vi "ControlShooter.vi"(1 "State":T2) -> (0 "To Shooter\nSolenoid Loop":T1=enum."Forward")   [LabVIEW 2013]
uses:
  typedefs/subStates.ctl
  <vilib>/Rock Robotics/WPI/Solenoid/WPI_SolenoidValue.ctl
  typedefs/fg_typedef.ctl
  <vilib>/Rock Robotics/WPI/Solenoid/WPI_SolenoidGetEnum.vi
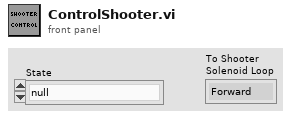
[diagram p1: front panel]
types:
  T1 = typedef "WPI_SolenoidValue.ctl" = enum16{"Off", "On", "Forward", "Reverse"}
  T2 = typedef "subStates.ctl" = enum16{"null", "wait", "driver control", "auto", "manual override", "hold position", "rotate", "pickup", "pass", "load", "goto shoot", "shoot", "cancel", "end"}
  T3 = typedef "fg_typedef.ctl" = enum16{"Get", "Set"}
  T4 = typedef "WPI_DigitalInputDevRef.ctl" = cluster{"DevStatus":errorcluster, "DIO Channel":T5, "Digital Module":T6}
  T5 = typedef "FPGA_DIOChannel.ctl" = enum8{"DIO 1", "DIO 2", "DIO 3", "DIO 4", "DIO 5", "DIO 6", "DIO 7", "DIO 8", "DIO 9", "DIO 10", "DIO 11", "DIO 12", "DIO 13", "DIO 14", "Invalid"}
  T6 = typedef "FPGA_TypedefDigitalModule.ctl" = enum16{"Digital Module 1", "Digital Module 2"}
  T7 = typedef "WPI_SolenoidDevRef.ctl" = cluster{"DevStatus":errorcluster, "Solenoid Module":T8, "Forward Solenoid Channel":T9, "Reverse Solenoid Channel":T9}
  T8 = typedef "FPGA_TypedefSolenoidModule.ctl" = enum16{"Solenoid Module 1", "Solenoid Module 2"}
  T9 = typedef "WPI_SolenoidChannel.ctl" = enum8{"Solenoid 1", "Solenoid 2", "Solenoid 3", "Solenoid 4", "Solenoid 5", "Solenoid 6", "Solenoid 7", "Solenoid 8", "Invalid"}
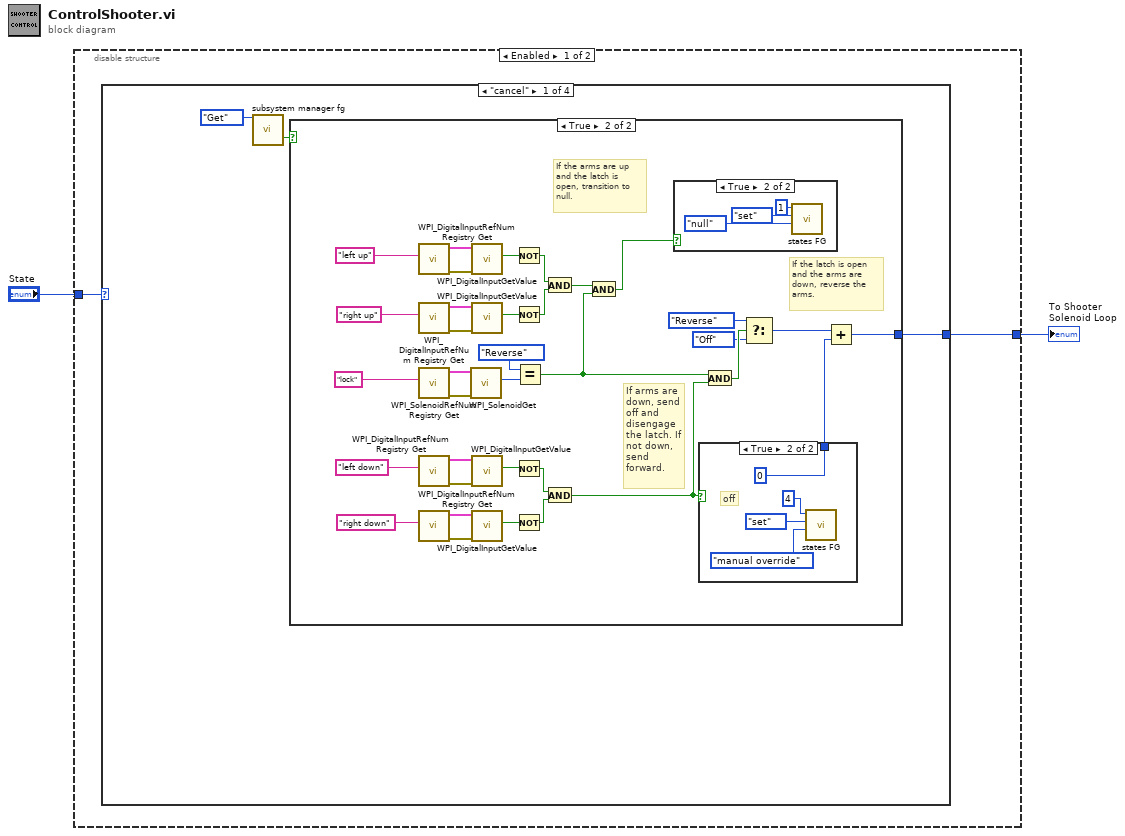
[diagram p0: block diagram]
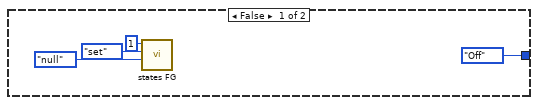
[diagram p2: hidden frame]
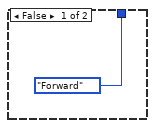
[diagram p4: hidden frame]
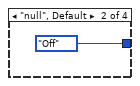
[diagram p5: hidden frame]
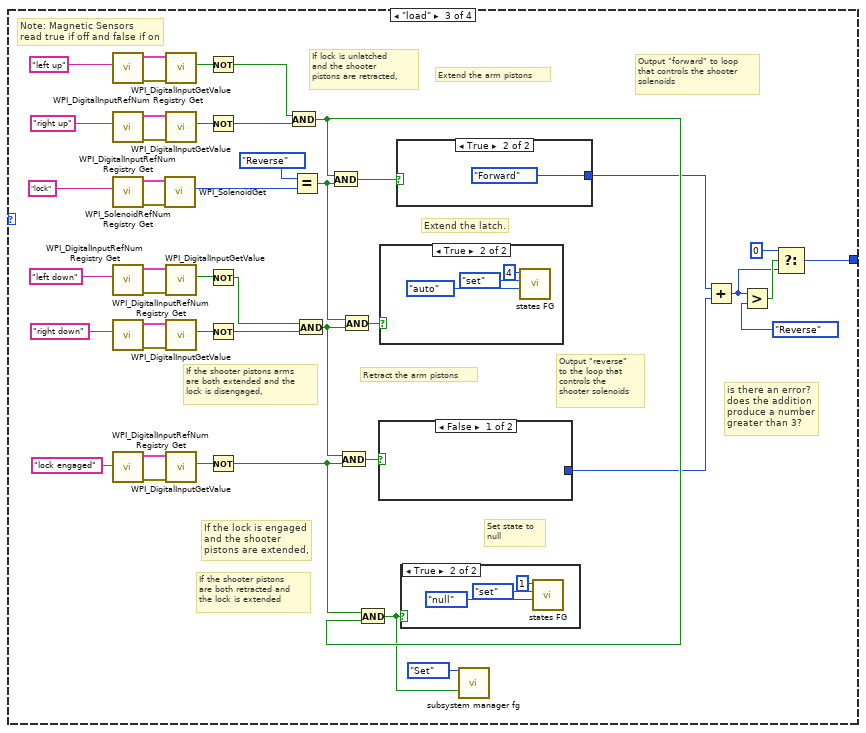
[diagram p6: hidden frame]
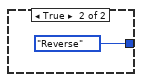
[diagram p8: hidden frame]
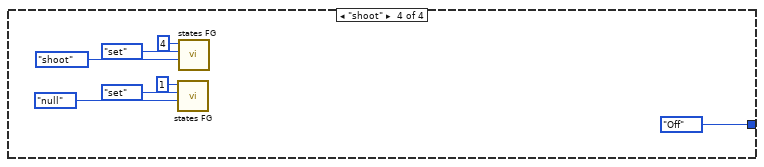
[diagram p11: hidden frame]
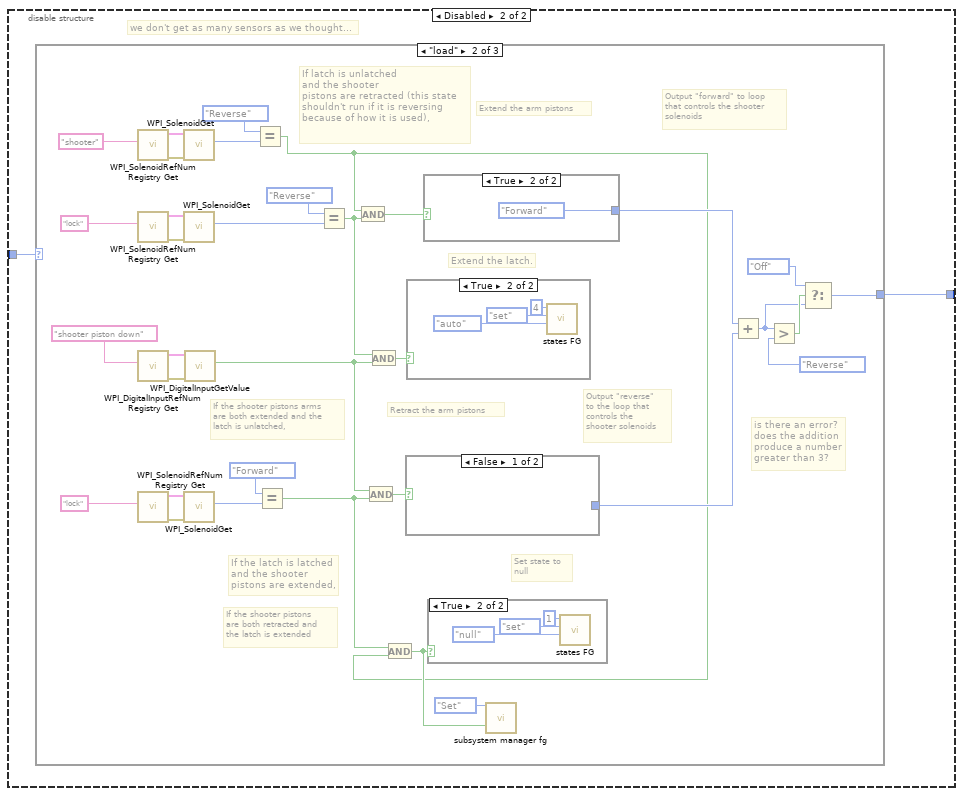
[diagram p12: hidden frame]
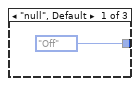
[diagram p13: hidden frame]
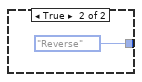
[diagram p15: hidden frame]
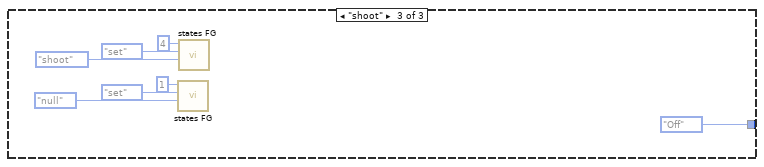
[diagram p18: hidden frame]
diagram:
  n1 = disable-structure shown="Enabled" {
    disable-tunnel: "State" -> [w4 w117]
    disable-tunnel: [w3 w116] -> w1
    frame Enabled {
      n2 = case shown="\"cancel\"" w4 {
        tunnel: [w5 WPI_SolenoidValue."Off" ("To Shooter\nSolenoid Loop") w72 WPI_SolenoidValue."Off" ("To Shooter\nSolenoid Loop")] -> w3
        frame "cancel" {
          n3 = call "subsystem manager fg.vi"("Menu"=fg_typedef."Get") -> ("Shooter Cocked"=w6:bool)  [unwired: 14 in, 4 out]
          n4 = case shown="True" w6 {
            tunnel: [WPI_SolenoidValue."Off" ("To Shooter\nSolenoid Loop") w15] -> w5
            frame False {
              n5 = call "states FG.vi"("subState in"=subStates."null", "menu (get)"=enum16{"set", "get"}."set", "Loop ID"=1) -> ()  [unwired: 5 in, 4 out]
            }
            frame True {
              # "If the arms are up\nand the latch is\nopen, transition to\nnull."
              # "If the latch is open\nand the arms are\ndown, reverse the\narms."
              # "If arms are\ndown, send\noff and\ndisengage\nthe latch. If\nnot down,\nsend\nforward."
              n6 = call <vilib>:"WPI_DigitalInputRefNum Registry Get.vi"("refnum name"="left up") -> ("error out"=w33:errorcluster, "DigitalInputDevRef"=w32:T4)  [unwired: 9 in]
              n7 = call <vilib>:"WPI_DigitalInputRefNum Registry Get.vi"("refnum name"="right up") -> ("error out"=w30:errorcluster, "DigitalInputDevRef"=w29:T4)  [unwired: 9 in]
              n8 = call <vilib>:"WPI_SolenoidRefNum Registry Get.vi"("refnum name"="lock") -> ("error out"=w26:errorcluster, "SolenoidDevRef"=w27:T7)  [unwired: 9 in]
              n9 = call <vilib>:"WPI_DigitalInputRefNum Registry Get.vi"("refnum name"="left down") -> ("error out"=w36:errorcluster, "DigitalInputDevRef"=w35:T4)  [unwired: 9 in]
              n10 = call <vilib>:"WPI_DigitalInputRefNum Registry Get.vi"("refnum name"="right down") -> ("error out"=w39:errorcluster, "DigitalInputDevRef"=w38:T4)  [unwired: 9 in]
              n11 = call-poly <vilib>:"WPI_SolenoidGet.vi"("error in (no error)"=w26, "SolenoidDevRef"=w27) -> ("Value"=w45:T1)  [unwired: 7 in, 2 out]
              n12 = call <vilib>:"WPI_DigitalInputGetValue.vi"("error in (no error)"=w33, "DigitalInputDevRef"=w32) -> ("Value"=w44:bool)  [unwired: 7 in, 2 out]
              n13 = call <vilib>:"WPI_DigitalInputGetValue.vi"("error in (no error)"=w30, "DigitalInputDevRef"=w29) -> ("Value"=w43:bool)  [unwired: 7 in, 2 out]
              n14 = call <vilib>:"WPI_DigitalInputGetValue.vi"("error in (no error)"=w36, "DigitalInputDevRef"=w35) -> ("Value"=w42:bool)  [unwired: 7 in, 2 out]
              n15 = call <vilib>:"WPI_DigitalInputGetValue.vi"("error in (no error)"=w39, "DigitalInputDevRef"=w38) -> ("Value"=w41:bool)  [unwired: 7 in, 2 out]
              n16 = Not(x=w44) -> (.not. x?=w24:bool)
              n17 = Not(x=w43) -> (.not. x?=w25:bool)
              n18 = Not(x=w42) -> (.not. x?=w22:bool)
              n19 = Not(x=w41) -> (.not. x?=w23:bool)
              n20 = Equal?(x=WPI_SolenoidValue."Reverse", y=w45) -> (x = y?=w13:bool)
              n21 = And(x=w24, y=w25) -> (x .and. y?=w14:bool)
              n22 = And(x=w22, y=w23) -> (x .and. y?=w21:bool)
              n23 = And(x=w14, y=w13) -> (x .and. y?=w12:bool)
              n24 = case shown="True" w12 {
                frame False {
                }
                frame True {
                  n25 = call "states FG.vi"("subState in"=subStates."null", "menu (get)"=enum16{"set", "get"}."set", "Loop ID"=1) -> ()  [unwired: 5 in, 4 out]
                }
              }
              n26 = case shown="True" w21 {
                tunnel: [WPI_SolenoidValue."Forward" ("To Shooter\nSolenoid Loop") 0] -> w20
                frame False {
                }
                frame True {
                  # "off"
                  n27 = call "states FG.vi"("subState in"=subStates."manual override", "menu (get)"=enum16{"set", "get"}."set", "Loop ID"=4) -> ()  [unwired: 5 in, 4 out]
                }
              }
              n28 = And(x=w13, y=w21) -> (x .and. y?=w19:bool)
              n29 = Select(t=WPI_SolenoidValue."Reverse" ("To Shooter\nSolenoid Loop"), s=w19, f=WPI_SolenoidValue."Off") -> (s? t:f=w17:T1)
              n30 = Add(x=w17, y=w20) -> (x+y=w15:i32)
            }
          }
        }
        frame "null", Default {
        }
        frame "load" {
          # "Note: Magnetic Sensors\nread true if off and false if on"
          # "is there an error?\ndoes the addition\nproduce a number \ngreater than 3?"
          # "Output \"reverse\"\nto the loop that\ncontrols the\nshooter solenoids"
          # "Output \"forward\" to loop\nthat controls the shooter\nsolenoids"
          # "Set state to\nnull"
          # "If the shooter pistons\nare both retracted and\nthe lock is extended"
          # "If the lock is engaged\nand the shooter\npistons are extended,"
          # "Retract the arm pistons"
          # "If lock is unlatched\nand the shooter\npistons are retracted,"
          # "Extend the latch."
          # "If the shooter pistons arms\nare both extended and the\nlock is disengaged,"
          # "Extend the arm pistons"
          n31 = call <vilib>:"WPI_DigitalInputRefNum Registry Get.vi"("refnum name"="left up") -> ("error out"=w91:errorcluster, "DigitalInputDevRef"=w92:T4)  [unwired: 9 in]
          n32 = call <vilib>:"WPI_DigitalInputRefNum Registry Get.vi"("refnum name"="right up") -> ("error out"=w94:errorcluster, "DigitalInputDevRef"=w95:T4)  [unwired: 9 in]
          n33 = call <vilib>:"WPI_SolenoidRefNum Registry Get.vi"("refnum name"="lock") -> ("error out"=w100:errorcluster, "SolenoidDevRef"=w99:T7)  [unwired: 9 in]
          n34 = call <vilib>:"WPI_DigitalInputRefNum Registry Get.vi"("refnum name"="left down") -> ("error out"=w86:errorcluster, "DigitalInputDevRef"=w87:T4)  [unwired: 9 in]
          n35 = call <vilib>:"WPI_DigitalInputRefNum Registry Get.vi"("refnum name"="right down") -> ("error out"=w83:errorcluster, "DigitalInputDevRef"=w84:T4)  [unwired: 9 in]
          n36 = call <vilib>:"WPI_DigitalInputRefNum Registry Get.vi"("refnum name"="lock engaged") -> ("error out"=w66:errorcluster, "DigitalInputDevRef"=w67:T4)  [unwired: 9 in]
          n37 = call-poly <vilib>:"WPI_SolenoidGet.vi"("error in (no error)"=w100, "SolenoidDevRef"=w99) -> ("Value"=w97:T1)  [unwired: 7 in, 2 out]
          n38 = call <vilib>:"WPI_DigitalInputGetValue.vi"("error in (no error)"=w91, "DigitalInputDevRef"=w92) -> ("Value"=w57:bool)  [unwired: 7 in, 2 out]
          n39 = call <vilib>:"WPI_DigitalInputGetValue.vi"("error in (no error)"=w94, "DigitalInputDevRef"=w95) -> ("Value"=w59:bool)  [unwired: 7 in, 2 out]
          n40 = call <vilib>:"WPI_DigitalInputGetValue.vi"("error in (no error)"=w86, "DigitalInputDevRef"=w87) -> ("Value"=w61:bool)  [unwired: 7 in, 2 out]
          n41 = call <vilib>:"WPI_DigitalInputGetValue.vi"("error in (no error)"=w83, "DigitalInputDevRef"=w84) -> ("Value"=w63:bool)  [unwired: 7 in, 2 out]
          n42 = call <vilib>:"WPI_DigitalInputGetValue.vi"("error in (no error)"=w66, "DigitalInputDevRef"=w67) -> ("Value"=w65:bool)  [unwired: 7 in, 2 out]
          n43 = Not(x=w57) -> (.not. x?=w56:bool)
          n44 = Not(x=w59) -> (.not. x?=w58:bool)
          n45 = Not(x=w61) -> (.not. x?=w60:bool)
          n46 = Not(x=w63) -> (.not. x?=w62:bool)
          n47 = Not(x=w65) -> (.not. x?=w64:bool)
          n48 = And(x=w56, y=w58) -> (x .and. y?=w78:bool)
          n49 = Equal?(x=WPI_SolenoidValue."Reverse", y=w97) -> (x = y?=w79:bool)
          n50 = And(x=w60, y=w62) -> (x .and. y?=w80:bool)
          n51 = And(x=w78, y=w79) -> (x .and. y?=w89:bool)
          n52 = And(x=w80, y=w64) -> (x .and. y?=w81:bool)
          n53 = And(x=w79, y=w80) -> (x .and. y?=w88:bool)
          n54 = And(x=w64, y=w78) -> (x .and. y?=w69:bool)
          n55 = case shown="False" w81 {
            tunnel: [_ WPI_SolenoidValue."Reverse" ("Value")] -> w71
            frame False {
            }
            frame True {
            }
          }
          n56 = case shown="True" w88 {
            frame False {
            }
            frame True {
              n57 = call "states FG.vi"("subState in"=subStates."auto", "menu (get)"=enum16{"set", "get"}."set", "Loop ID"=4) -> ()  [unwired: 5 in, 4 out]
            }
          }
          n58 = case shown="True" w89 {
            tunnel: [_ WPI_SolenoidValue."Forward" ("Value")] -> w77
            frame False {
            }
            frame True {
            }
          }
          n59 = case shown="True" w69 {
            frame False {
            }
            frame True {
              n60 = call "states FG.vi"("subState in"=subStates."null", "menu (get)"=enum16{"set", "get"}."set", "Loop ID"=1) -> ()  [unwired: 5 in, 4 out]
            }
          }
          n61 = call "subsystem manager fg.vi"("Menu"=fg_typedef."Set", "Shooter Cocked"=w69) -> ()  [unwired: 13 in, 5 out]
          n62 = Add(x=w77, y=w71) -> (x+y=w74:u16)
          n63 = Greater?(x=w74, y=WPI_SolenoidValue."Reverse" ("Value")) -> (0:w75:bool)
          n64 = Select(t=0, s=w75, f=w74) -> (s? t:f=w72:i32)
        }
        frame "shoot" {
          n65 = call "states FG.vi"("subState in"=subStates."null", "menu (get)"=enum16{"set", "get"}."set", "Loop ID"=1) -> ()  [unwired: 5 in, 4 out]
          n66 = call "states FG.vi"("subState in"=subStates."shoot", "menu (get)"=enum16{"set", "get"}."set", "Loop ID"=4) -> ()  [unwired: 5 in, 4 out]
        }
      }
    }
    frame Disabled {
      # "we don't get as many sensors as we thought..."
      n67 = case shown="\"load\"" w117 {
        tunnel: [WPI_SolenoidValue."Off" ("To Shooter\nSolenoid Loop") w130 WPI_SolenoidValue."Off" ("To Shooter\nSolenoid Loop")] -> w116
        frame "null", Default {
        }
        frame "load" {
          # "is there an error?\ndoes the addition\nproduce a number \ngreater than 3?"
          # "Output \"reverse\"\nto the loop that\ncontrols the\nshooter solenoids"
          # "Output \"forward\" to loop\nthat controls the shooter\nsolenoids"
          # "Set state to\nnull"
          # "If the shooter pistons\nare both retracted and\nthe latch is extended"
          # "If the latch is latched\nand the shooter\npistons are extended,"
          # "Retract the arm pistons"
          # "If latch is unlatched\nand the shooter\npistons are retracted (this state shouldn't run if it is reversing because of how it is used),"
          # "Extend the latch."
          # "If the shooter pistons arms\nare both extended and the\nlatch is unlatched,"
          # "Extend the arm pistons"
          n68 = call <vilib>:"WPI_SolenoidRefNum Registry Get.vi"("refnum name"="shooter") -> ("error out"=w122:errorcluster, "SolenoidDevRef"=w123:T7)  [unwired: 9 in]
          n69 = call <vilib>:"WPI_SolenoidRefNum Registry Get.vi"("refnum name"="lock") -> ("error out"=w152:errorcluster, "SolenoidDevRef"=w151:T7)  [unwired: 9 in]
          n70 = call <vilib>:"WPI_DigitalInputRefNum Registry Get.vi"("refnum name"="shooter piston down") -> ("error out"=w144:errorcluster, "DigitalInputDevRef"=w145:T4)  [unwired: 9 in]
          n71 = call <vilib>:"WPI_SolenoidRefNum Registry Get.vi"("refnum name"="lock") -> ("error out"=w142:errorcluster, "SolenoidDevRef"=w141:T7)  [unwired: 9 in]
          n72 = call-poly <vilib>:"WPI_SolenoidGet.vi"("error in (no error)"=w122, "SolenoidDevRef"=w123) -> ("Value"=w124:T1)  [unwired: 7 in, 2 out]
          n73 = call-poly <vilib>:"WPI_SolenoidGet.vi"("error in (no error)"=w152, "SolenoidDevRef"=w151) -> ("Value"=w149:T1)  [unwired: 7 in, 2 out]
          n74 = call-poly <vilib>:"WPI_SolenoidGet.vi"("error in (no error)"=w142, "SolenoidDevRef"=w141) -> ("Value"=w139:T1)  [unwired: 7 in, 2 out]
          n75 = call <vilib>:"WPI_DigitalInputGetValue.vi"("error in (no error)"=w144, "DigitalInputDevRef"=w145) -> ("Value"=w126:bool)  [unwired: 7 in, 2 out]
          n76 = Equal?(x=WPI_SolenoidValue."Reverse", y=w124) -> (x = y?=w120:bool)
          n77 = Equal?(x=WPI_SolenoidValue."Forward", y=w139) -> (x = y?=w135:bool)
          n78 = Equal?(x=WPI_SolenoidValue."Reverse", y=w149) -> (x = y?=w136:bool)
          n79 = And(x=w120, y=w136) -> (x .and. y?=w147:bool)
          n80 = And(x=w126, y=w135) -> (x .and. y?=w137:bool)
          n81 = And(x=w136, y=w126) -> (x .and. y?=w146:bool)
          n82 = And(x=w135, y=w120) -> (x .and. y?=w127:bool)
          n83 = case shown="False" w137 {
            tunnel: [_ WPI_SolenoidValue."Reverse" ("Value")] -> w129
            frame False {
            }
            frame True {
            }
          }
          n84 = case shown="True" w146 {
            frame False {
            }
            frame True {
              n85 = call "states FG.vi"("subState in"=subStates."auto", "menu (get)"=enum16{"set", "get"}."set", "Loop ID"=4) -> ()  [unwired: 5 in, 4 out]
            }
          }
          n86 = case shown="True" w147 {
            tunnel: [_ WPI_SolenoidValue."Forward" ("Value")] -> w134
            frame False {
            }
            frame True {
            }
          }
          n87 = case shown="True" w127 {
            frame False {
            }
            frame True {
              n88 = call "states FG.vi"("subState in"=subStates."null", "menu (get)"=enum16{"set", "get"}."set", "Loop ID"=1) -> ()  [unwired: 5 in, 4 out]
            }
          }
          n89 = call "subsystem manager fg.vi"("Menu"=fg_typedef."Set", "Shooter Cocked"=w127) -> ()  [unwired: 13 in, 5 out]
          n90 = Add(x=w134, y=w129) -> (x+y=w131:u16)
          n91 = Greater?(x=w131, y=WPI_SolenoidValue."Reverse" ("Value")) -> (0:w132:bool)
          n92 = Select(t=WPI_SolenoidValue."Off" ("Value"), s=w132, f=w131) -> (s? t:f=w130:u16)
        }
        frame "shoot" {
          n93 = call "states FG.vi"("subState in"=subStates."null", "menu (get)"=enum16{"set", "get"}."set", "Loop ID"=1) -> ()  [unwired: 5 in, 4 out]
          n94 = call "states FG.vi"("subState in"=subStates."shoot", "menu (get)"=enum16{"set", "get"}."set", "Loop ID"=4) -> ()  [unwired: 5 in, 4 out]
        }
      }
    }
  }
  "To Shooter\nSolenoid Loop" <- w1
